vi "Read Exception Status Response.vi"(8 "error in":errorcluster, 10 "modbus data unit in":refnum<class "Modbus Data Unit.lvclass">) -> (0 "error out":errorcluster, 2 "Exception Status":u8)   [LabVIEW 2021, in "Master Function Definition.lvclass"]
doc: "Decodes the response generated by the read exception status function."
uses:
  Master Function Definition.lvclass
  Modbus Data Unit/Modbus Data Unit.lvclass
  Modbus Data Unit/Modbus Data Unit.lvclass/Modbus Data Unit.ctl
  Modbus Data Unit/Deconstruct PDU.vi
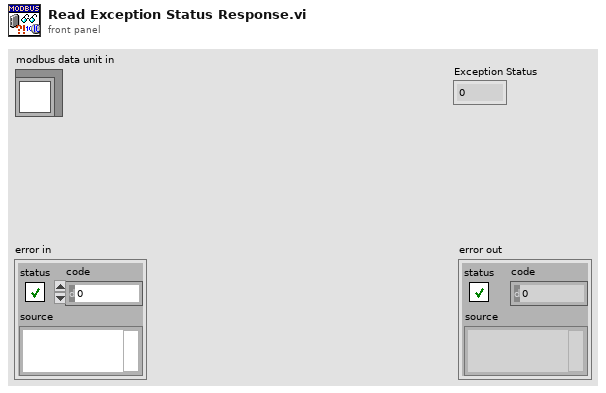
[diagram p1: front panel]
types:
  T1 = typedef "Modbus Data Unit.lvclass/Function.ctl" = u8
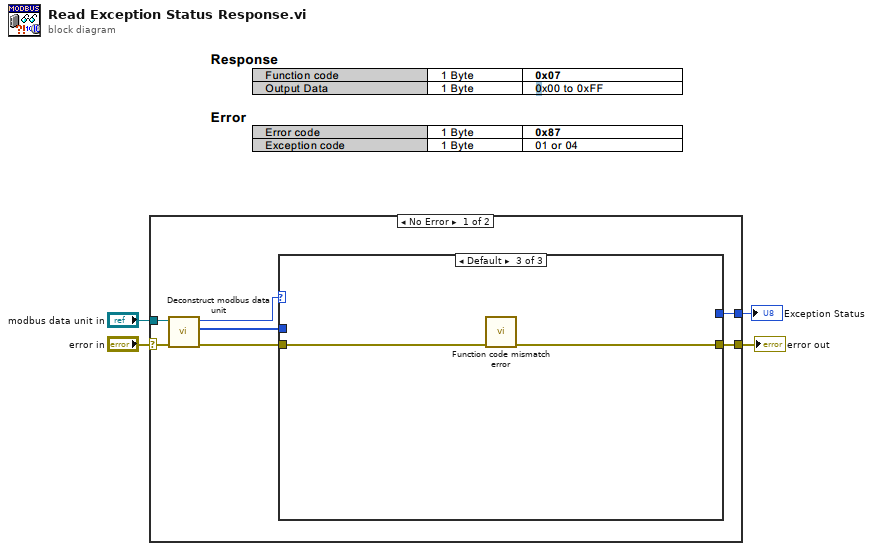
[diagram p0: block diagram]
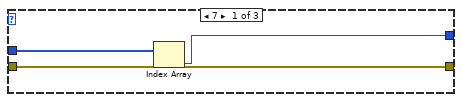
[diagram p2: hidden frame]
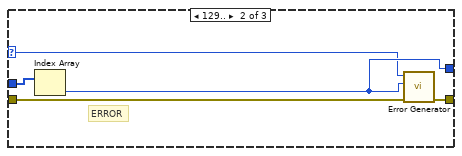
[diagram p3: hidden frame]
diagram:
  n1 = case shown="No Error" "error in" {
    selector: "error in" -> [w10 w22]
    tunnel: [w11 w22] -> w3
    tunnel: "modbus data unit in" -> [w8 _]
    tunnel: [w6 _] -> w1
    frame No Error {
      n2 = call "Deconstruct modbus data unit.vi"("error in"=w10, "modbus data unit in"=w8) -> ("error out"=w7:errorcluster, "data"=w9:u8[], "Function"=w5:T1)  [unwired: 7 in]
      n3 = case shown="Default" w5 {
        selector: w5 -> [_ w15 _]
        tunnel: w7 -> [w13 w17 w21]
        tunnel: w9 -> [w14 w19 _]
        tunnel: [w13 w18 w20] -> w11
        tunnel: [w12 w16 _] -> w6
        frame 7 {
          n4 = Index Array(array=w14) -> (element=w12:u8)  [unwired: 1 in]
        }
        frame 129.. {
          # "ERROR"
          n5 = Index Array(array=w19) -> (element=w16:u8)  [unwired: 1 in]
          n6 = call "Error Generator.vi"("error in"=w17, "data return (error code)"=w16, "function return"=w15) -> ("error out"=w18:errorcluster)  [unwired: 8 in]
        }
        frame Default {
          n7 = call "Function code mismatch error.vi"("error in (no error)"=w21) -> ("error out"=w20:errorcluster)  [unwired: 10 in]
        }
      }
    }
    frame Error {
    }
  }
  "error out" <- w3
  "Exception Status" <- w1
